vi "open picture(SubVI).vi"(9 "Picture number":i32, 10 "All Files in Dir":path[](array[path]), 11 "Categories":string[](array[string])) -> (2 "Category":i32, 3 "Image":T1)   [LabVIEW 2020]
uses:
  <vilib>/vision/Image Controls.llb/IMAQ Image.ctl
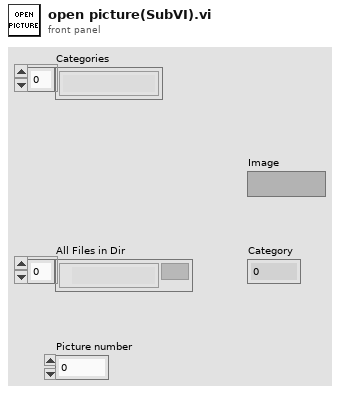
[diagram p1: front panel]
types:
  T1 = typedef "IMAQ Image.ctl" = refnum<image>
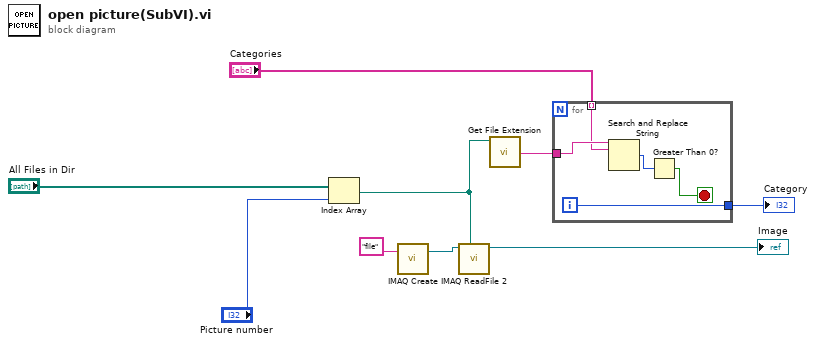
[diagram p0: block diagram]
diagram:
  n1 = Index Array(array="All Files in Dir", index="Picture number") -> (element=w4:path)
  n2 = call "IMAQ Create"("Image Name"="file") -> ("New Image"=w1:T1)  [unwired: 4 in, 1 out]
  n3 = call "IMAQ ReadFile 2"("File Path"=w4, "Image"=w1) -> ("Image Out"=→"Image":T1)  [unwired: 5 in, 4 out]
  n4 = call <vilib>:"Get File Extension.vi"("file"=w4) -> ("filename without extension"=w5:string)  [unwired: 6 in, 4 out]
  n5 = for {
    tunnel: "Categories" -> [w13] mode=indexing
    tunnel: w5 -> [w14]
    tunnel: [w10] -> w6
    i -> [w10]
    stop <- w11 stop-if-true
    n6 = Search and Replace String(input string=w14, search string=w13) -> (number of replacements=w12:i32)  [unwired: 6 in, 3 out]
    n7 = Greater Than 0?(x=w12) -> (x > 0?=w11:bool)
  }
  "Category" <- w6
